vi "_setOtherRef.vi"(7 "parentURL":string, 8 "error in (no error)":errorcluster, 9 "Name":string, 10 "Refnum":variant, 11 "TagDB in":T1) -> (0 "error out":errorcluster, 2 "Ref-Key":string, 3 "TagDB out":T1)   [LabVIEW 2017, in "TagDB RefManager.lvlib"]
uses:
  TagDB RefManager.lvlib
  <userlib>/_NEVSTOP/TagDB/Typedef/TagDB.ctl
  ad25227d-9584-495d-a87b-e5128456ff42.vi
  87945a8b-64f7-4dda-81c3-3593ac262b7b.vi
  <userlib>/_NEVSTOP/TagDB/_Support/DataAccess/data-Write.vi
  <userlib>/_NEVSTOP/TagDB/_Support/DataAccess/TagDB Ref to DVR.vi
  <userlib>/_NEVSTOP/TagDB/_Support/DataAccess/_NameCacher.vi
  <userlib>/_NEVSTOP/TagDB/_Support/DataAccess/_datatypeChecker.vi
  <vilib>/Utility/Data Type/Get Type Information.vi
  <userlib>/_NEVSTOP/TagDB/_Support/Error/_[error50000]Invalid DB REF.vi
  <userlib>/_NEVSTOP/TagDB/TagDB.lvlib
  <vilib>/Utility/Data Type/NI_Data Type.lvlib
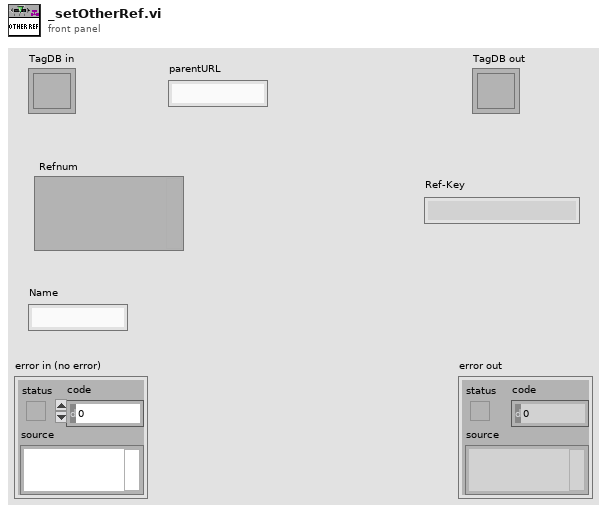
[diagram p1: front panel]
types:
  T1 = typedef "TagDB.lvlib/TagDB.ctl" = refnum<k1>
  T2 = typedef "NI_Data Type.lvlib/Refnum Type.ctl" = enum16{"NotARefnum", "UnknownRefnum", "Generic", "Datalog", "ByteStream", "Device", "Occurence", "TCPNetConnection", "Auto", "Menu", "Imaq", "Hardware", "DataSocket", "Visa", "IVI", "UDPNetConnection", "Notifier", "Queue", "Irda", "EventReg", "DotNet", "UserEvent", "Callback", "UNUSED_EMPTY_POSITION", "BlueToothNetConnection", "LVObjApp", "LVObjVI", "LVObjUnknown", "GenericClass", "UserDefinedRefnumTag", "DataValue", "RT FIFO", "TDMS File"}
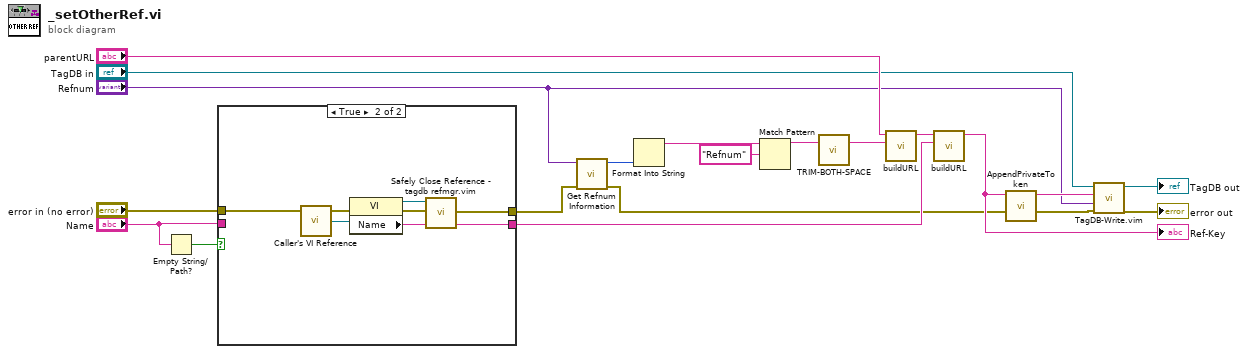
[diagram p0: block diagram]
diagram:
  n1 = Empty String/Path?(string/path="Name") -> (empty?=w19:bool)
  n2 = case shown="True" w19 {
    tunnel: [w21 w23] -> w11
    tunnel: "Name" -> [w21 _]
    tunnel: "error in (no error)" -> [w20 w25]
    tunnel: [w20 w24] -> w2
    frame False {
    }
    frame True {
      n3 = call "Caller's VI Reference.vi"("error in (no error)"=w25) -> ("error out"=w28:errorcluster, "Caller's VI Reference"=w27:refnum<vi>)  [unwired: 5 in]
      n4 = property on="Property Node" class="VI"(reference=w27, error in=w28) -> (reference out=w26:refnum<vi>, error out=w22:errorcluster, "Name"=w23:string)
      n5 = call "Safely Close Reference - tagdb refmgr.vim"("error in (no error)"=w22, "Reference"=w26) -> ("error out"=w24:errorcluster)  [unwired: 9 in]
    }
  }
  n6 = call <vilib>:"Get Refnum Information.vi"("error in (no error)"=w2, "Variant"="Refnum") -> ("error out"=w1:errorcluster, "Reference Type"=w3:T2)  [unwired: 6 in, 2 out]
  n7 = Format Into String(w3) -> (resulting string=w14:string)  [unwired: 3 in, 1 out]
  n8 = Match Pattern(string=w14, regular expression="Refnum") -> (before substring=w12:string)  [unwired: 1 in, 3 out]
  n9 = call <userlib>:"TRIM-BOTH-SPACE.vi"("name in"=w12) -> ("name out"=w15:string)  [unwired: 2 in]
  n10 = call <userlib>:"buildURL.vi"("DataName"=w15, "parentURL"="parentURL") -> ("DataURL"=w16:string)  [unwired: 9 in]
  n11 = call <userlib>:"buildURL.vi"("DataName"=w11, "parentURL"=w16) -> ("DataURL"=w4:string)  [unwired: 9 in]
  "Ref-Key" <- w4
  n12 = call <userlib>:"AppendPrivateToken.vi"("DataURL"=w4) -> ("String"=w7:string)  [unwired: 10 in]
  n13 = call "TagDB-Write.vim"("error in (no error)"=w1, "Value"="Refnum", "tag"=w7, "TagDB"="TagDB in") -> ("error out"=→"error out":errorcluster, "TagDB(dup)"=→"TagDB out":T1)  [unwired: 5 in, 1 out]
